vi "Add Topic Subscriber.vi"(8 "error in (no error)":errorcluster, 10 "Subscription Policy":T1, 11 "Topic in":refnum<class "Topic.lvclass">) -> (0 "error out":errorcluster, 3 "Topic out":refnum<class "Topic.lvclass">)   [LabVIEW 2015, in "Mediator.lvlib" / "Topic.lvclass"]
doc: "<License>\nCopyright © 2017 Composed Systems, LLC | All rights reserved\nwww.composed.io\n\nAuthor: Ethan Stern <ethan.stern@composed.io>\n\nThis software is provided \"AS IS\" WITHOUT WARRANTIES, either express or implied, AND IS FOR EDUCATIONAL PURPOSES ONLY.\n</License>"
uses:
  Topic.lvclass
  IMediator/ISubscriptionPolicy/ISubscriptionPolicy Reference.ctl
  IMediator/ISubscriptionPolicy/ISubscriptionPolicy.lvclass
  Topic.lvclass/Topic.ctl
  <vilib>/Utility/error.llb/Trim Whitespace.vi
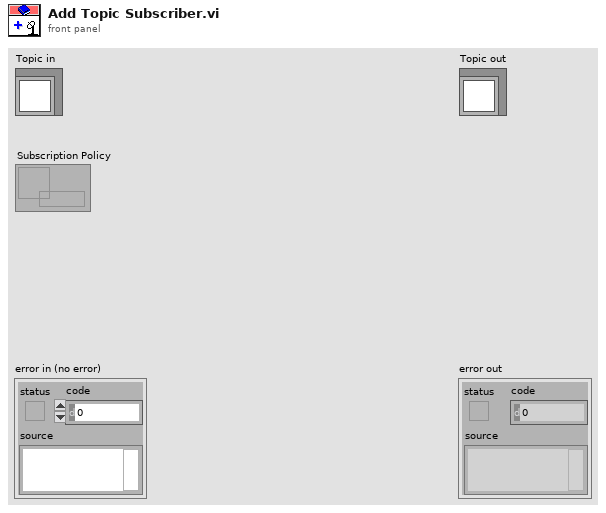
[diagram p1: front panel]
types:
  T1 = typedef "IMediator.lvlib/ISubscriptionPolicy.lvclass/ISubscriptionPolicy Reference.ctl" = refnum<data-value>
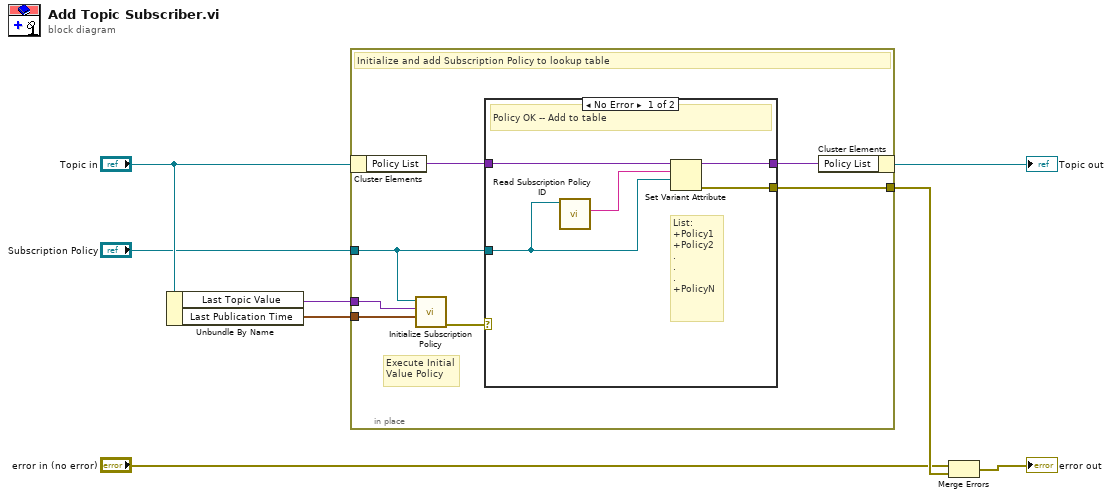
[diagram p0: block diagram]
diagram:
  n1 = Unbundle By Name("Topic in") -> ("Last Topic Value"=w4:variant, "Last Publication Time"=w3:timestamp)
  n2 = in-place {
    in-place-border: [w13] -> w8
    in-place-border: "Subscription Policy" -> [w9]
    in-place-border: w4 -> [w12]
    in-place-border: w3 -> [w10]
    # "Execute Initial\nValue Policy"
    # "Initialize and add Subscription Policy to lookup table"
    n3 = in-place-cluster #1("Topic in") -> ("Policy List"=w15:variant)
    n4 = call "Initialize Subscription Policy.vi"("Last Publish Time"=w10, "Last Topic Value"=w12, "Subscription Policy"=w9) -> ("Error Out (Do Not Subscribe?)"=w11:errorcluster)  [unwired: 8 in]
    n5 = case shown="No Error" w11 {
      tunnel: w15 -> [w18 w21]
      tunnel: [w20 w21] -> w14
      tunnel: [w19 _] -> w13
      tunnel: w9 -> [w16 _]
      frame No Error {
        # "List:\n+Policy1\n+Policy2\n.\n.\n.\n+PolicyN"
        # "Policy OK -- Add to table"
        n6 = call "Read Subscription Policy ID.vi"("SubscriptionPolicy"=w16) -> ("Policy ID"=w17:string)  [unwired: 10 in]
        n7 = Set Variant Attribute(Variant=w18, name=w17, value=w16) -> (Variant out=w20:variant, error out=w19:errorcluster)  [unwired: 1 in, 1 out]
      }
      frame Error {
        # "Policy is not valid --\nDo not add to table"
        # "A rough start -- Discard request"
      }
    }
    n8 = in-place-cluster #1("Policy List"=w14) -> (→"Topic out":refnum<class "Topic.lvclass">)
  }
  n9 = Merge Errors("error in (no error)", w8) -> (→"error out":errorcluster)
